vi "simpleReader.vi"() -> ()   [LabVIEW 2022 SP3]
uses:
  ActiveMQBroker/ActiveMQBroker.lvclass
panel:
  in  "Path":path=path "C:/VIs/RIMAS/instrument control/TCS/ActiveMQ/ActiveMQ_dll"
  out "messages received":string[][](table)
  in  "stopReader":bool
  in  "topic":string="testTopic"
  in  "port":string="61616"
  in  "host":string="localhost"
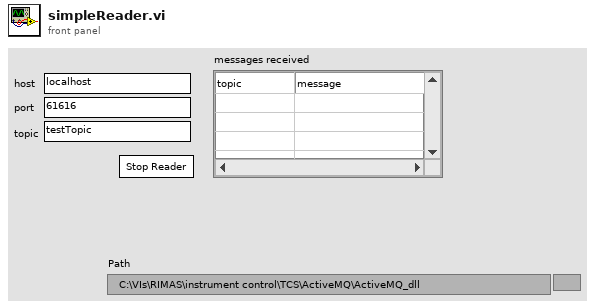
[diagram p1: front panel]
types:
  T1 = enum32{"invalid app kind", "Development System", "Run Time System", "Student Edition", "Embedded LabVIEW", "Evaluation", "Custom"}
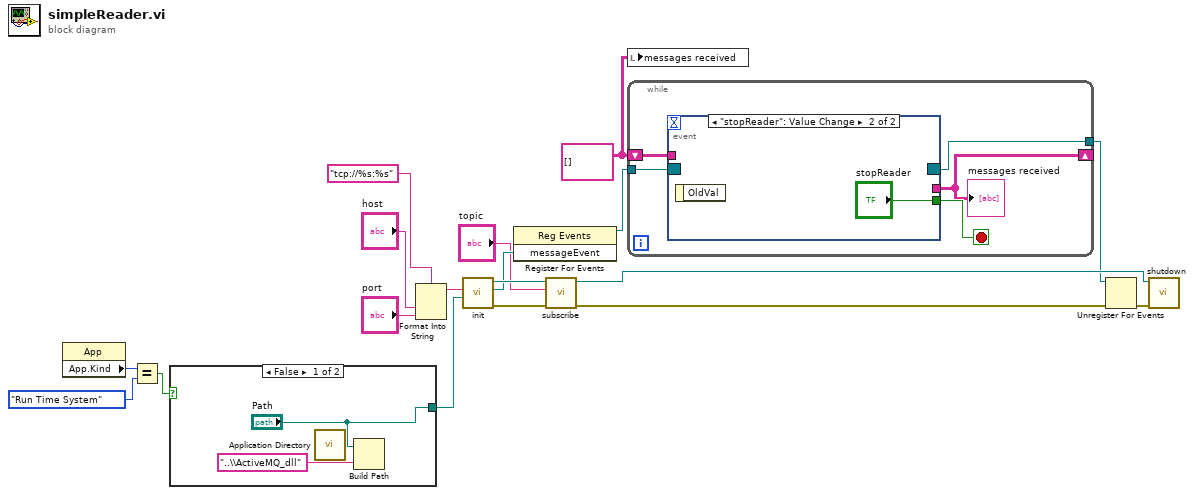
[diagram p0: block diagram]
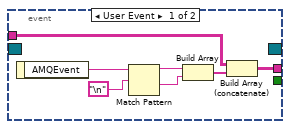
[diagram p2: hidden frame]
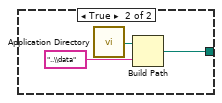
[diagram p3: hidden frame]
diagram:
  w1 = string[][] [] ("messages received")
  n1 = property class="App"() -> ("App.Kind"=w13:T1)  [unwired: 2 in, 2 out]
  n2 = Equal?(x=w13, y=T1."Run Time System") -> (x = y?=w11:bool)
  n3 = case shown="False" w11 {
    tunnel: ["Path" w21] -> w18
    frame False {
      n4 = call <vilib>:"Application Directory.vi"() -> ()  [unwired: 1 out]
      n5 = Build Path(base path="Path", name or relative path="..\\ActiveMQ_dll") -> ()  [unwired: 1 out]
    }
    frame True {
      n6 = call <vilib>:"Application Directory.vi"() -> ("Application Directory"=w23:path)
      n7 = Build Path(base path=w23, name or relative path="..\\data") -> (appended path=w21:path)
    }
  }
  n8 = Format Into String(format string="tcp://%s:%s", "host", "port") -> (resulting string=w7:string)  [unwired: 2 in, 1 out]
  n9 = call "init.vi"("activeMQ_dll_directory"=w18, "brokerConnectionString"=w7) -> ("error out"=w17:errorcluster, "messageEvent"=w15:refnum<user-event>, "ActiveMQBroker out"=w16:refnum<class "ActiveMQBroker.lvclass">)  [unwired: 7 in]
  n10 = register-events(w15) -> (reference out=w6:refnum<event-registration>)  [unwired: 2 in, 1 out]
  n11 = call-dynamic "subscribe.vi"("error in (no error)"=w17, "source"="topic", "ActiveMQBroker in"=w16) -> ("error out"=w3:errorcluster, "ActiveMQBroker out"=w14:refnum<class "ActiveMQBroker.lvclass">)  [unwired: 7 in]
  n12 = local write "messages received"(w1) -> ()
  n13 = while {
    tunnel: w6 -> [w28]
    tunnel: [w27] -> w5
    shift-right: [w24] -> _
    shift-left: w1 -> [w26]
    stop <- w25 stop-if-true
    n14 = event shown="[1] \"stopReader\": Value Change" {
      selector: w28 -> [_ _]
      dyn-events: [_ _] -> w27
      timeout: _ -> [_ _]
      tunnel: [w30 _] -> w24
      tunnel: w26 -> [w35 _]
      tunnel: [_ "stopReader"] -> w25
      event User Event {
        n15 = event-data() -> ("AMQEvent"=w34:string)  [unwired: 1 in]
        n16 = Match Pattern(string=w34, regular expression="\n") -> (before substring=w33:string, after substring=w32:string)  [unwired: 1 in, 2 out]
        n17 = Build Array(w33, w32) -> (w31:string[])
        n18 = Build Array (concatenate)(w35, w31) -> (w30:string[][])
      }
      event "stopReader": Value Change {
        n19 = event-data() -> ()  [unwired: 1 in, 1 out]
      }
    }
    "messages received" <- w24
  }
  n20 = Unregister For Events(event registration refnum=w5, error in=w3) -> (error out=w4:errorcluster)
  n21 = call-dynamic "shutdown.vi"("error in (no error)"=w4, "ActiveMQBroker in"=w14) -> ()  [unwired: 8 in, 2 out]
